vi "GetTimeArrayAsDouble.vi"(11 "Waveform":waveform(dbl)) -> (3 "Time Array":dbl[](array[numeric]))   [LabVIEW 2019]
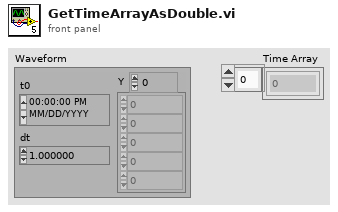
[diagram p1: front panel]
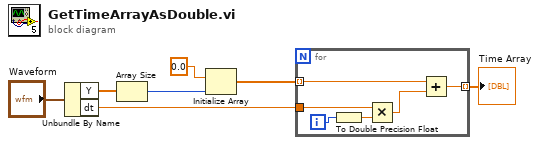
[diagram p0: block diagram]
diagram:
  n1 = Unbundle By Name("Waveform") -> ("Y"=w3:dbl[], "dt"=w4:dbl)
  n2 = Array Size(array=w3) -> (size(s)=w1:i32)
  n3 = Initialize Array(0.0, w1) -> (w6:dbl[])
  n4 = for {
    tunnel: w6 -> [w9] mode=indexing
    tunnel: w4 -> [w12]
    tunnel: [w8] -> w7 mode=indexing
    i -> [w13]
    n5 = To Double Precision Float(number=w13) -> (double precision float=w11:dbl)
    n6 = Multiply(x=w12, y=w11) -> (x*y=w10:dbl)
    n7 = Add(x=w9, y=w10) -> (x+y=w8:dbl)
  }
  "Time Array" <- w7
